vi "Database Recordset Fetch All.vi"(8 "error in (no error)":errorcluster caption="错误输入（无错误）", 11 "Database Recordset 输入":refnum<class "Database Recordset.lvclass"> caption="DNL_LabVIEW Object in") -> (0 "error out":errorcluster caption="错误输出", 1 "Data":variant[][](array[variant]), 3 "Database Recordset 输出":refnum<class "Database Recordset.lvclass"> caption="DNL_LabVIEW Object out")   [LabVIEW 2011, in "Database Recordset.lvclass"]
uses:
  Database Recordset.lvclass
  Database Recordset.lvclass/Database Recordset.ctl
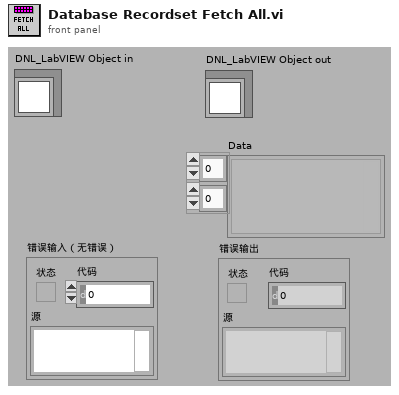
[diagram p1: front panel]
types:
  T1 = typedef "NI_Database_API.lvlib/DB Tools Cursor Type.ctl" = enum16{"forward-only", "keyset", "dynamic", "static"}
  T2 = cluster{"column count":i32, "record index":i32, "record count":i32, "bof?":bool, "eof?":bool, "cursor type":T1, "cache size":i32, "state":enum16{"closed", "open"}}
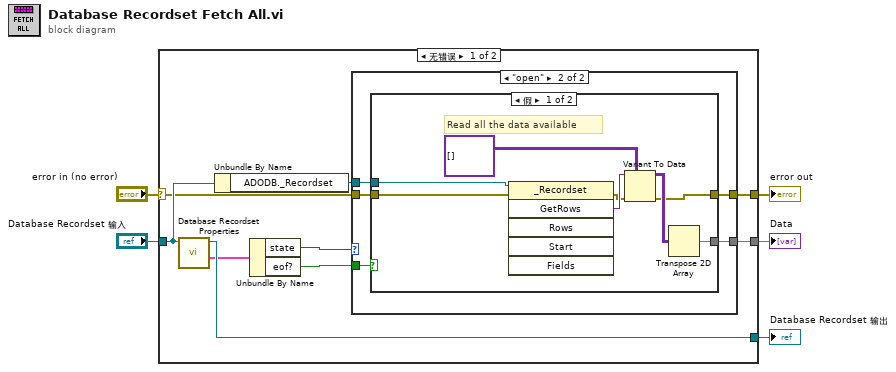
[diagram p0: block diagram]
diagram:
  n1 = case shown="无错误" "error in (no error)" {
    selector: "error in (no error)" -> [w8 w31]
    tunnel: [w7 w31] -> w4
    tunnel: [w14 w30] -> w2
    tunnel: "Database Recordset 输入" -> [w10 w30]
    tunnel: [w6 _] -> w1
    frame No Error {
      n2 = call "Database Recordset Properties.vi"("Database Recordset 输入"=w10) -> ("recordset properties"=w13:T2, "Database Recordset 输出"=w14:refnum<class "Database Recordset.lvclass">)  [unwired: 8 in, 1 out]
      n3 = Unbundle By Name(w10) -> ("ADODB._Recordset"=w9:refnum<k7>)
      n4 = Unbundle By Name(w13) -> ("state"=w12:enum16{"closed", "open"}, "eof?"=w11:bool)
      n5 = case shown="\"open\"" w12 {
        tunnel: [w15 w20] -> w7
        tunnel: [_ w19] -> w6
        tunnel: w11 -> [_ w18]
        tunnel: w9 -> [_ w17]
        tunnel: w8 -> [w15 w16]
        frame "closed" {
        }
        frame "open" {
          n6 = case shown="假" w18 {
            tunnel: [w25 w29] -> w20
            tunnel: [w24 _] -> w19
            tunnel: w17 -> [w22 _]
            tunnel: w16 -> [w21 w29]
            frame False {
              # "Read all the data available"
              n7 = invoke class="_Recordset" method="GetRows"(reference=w22, error in=w21) -> (error out=w26:errorcluster, "GetRows"=w27:variant)  [unwired: 4 in, 4 out]
              n8 = Variant To Data(error in=w26, type=variant[][] [], Variant=w27) -> (data=w28:variant[][], error out=w25:errorcluster)
              n9 = Transpose 2D Array(2D array=w28) -> (transposed array=w24:variant[][])
            }
            frame True {
            }
          }
        }
      }
    }
    frame Error {
    }
  }
  "error out" <- w4
  "Database Recordset 输出" <- w2
  "Data" <- w1
